vi "create tcp server.vi"(8 "error in":errorcluster, 10 "max allowed":i32=-1, 11 "conn string":string="localhost:5555/servicename") -> (0 "error out":errorcluster, 3 "TCP server out":refnum<class "TCP server.lvclass">)   [LabVIEW 2015, in "TCP server.lvclass"]
uses:
  TCP server.lvclass
  server/connection server.lvclass
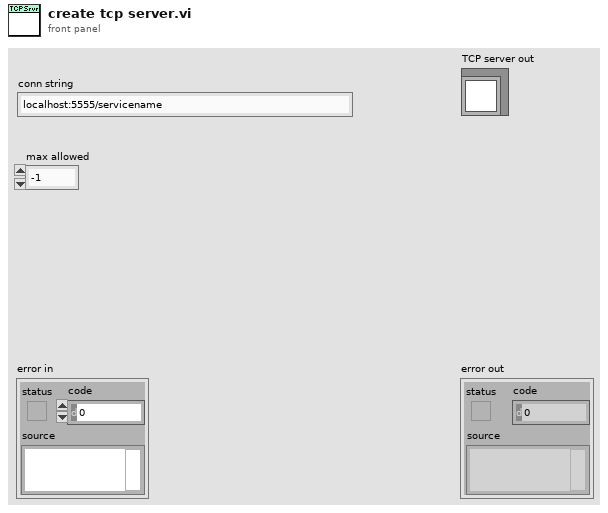
[diagram p1: front panel]
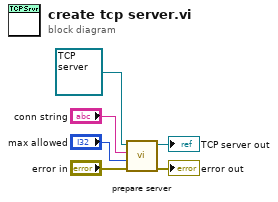
[diagram p0: block diagram]
diagram:
  n1 = call "prepare server.vi"("error in"="error in", "max allowed"="max allowed", "connection string"="conn string", "connection server in"=refnum<class "TCP server.lvclass"> refnum ("TCP server out 2")) -> ("error out"=→"error out":errorcluster, "connection server out"=→"TCP server out":refnum<class "TCP server.lvclass">)  [unwired: 6 in]
